vi "CRYGet Tab Reference.vi"(10 "Label Name":string, 11 "VI Refnum":refnum<vi>) -> (1 "Find?":bool, 2 "Tab Ref Out":refnum<vi>, 3 "VI Refnum Out":refnum<vi>)   [LabVIEW 2013]
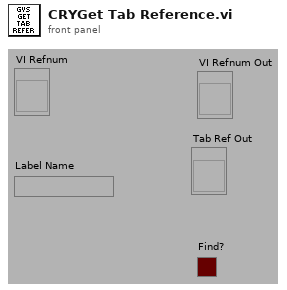
[diagram p1: front panel]
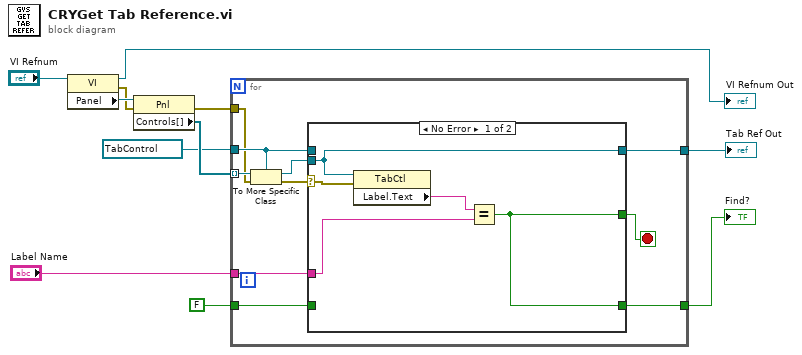
[diagram p0: block diagram]
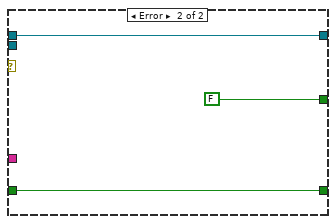
[diagram p2: hidden frame]
diagram:
  n1 = property class="VI"(reference="VI Refnum") -> (reference out=→"VI Refnum Out":refnum<vi>, error out=w2:errorcluster, "Panel"=w6:refnum<vi>)  [unwired: 1 in]
  n2 = property class="Pnl"(reference=w6, error in=w2) -> (error out=w1:errorcluster, "Controls[]"=w10:refnum<vi>[])  [unwired: 1 out]
  n3 = for {
    tunnel: w10 -> [w21] mode=indexing
    tunnel: [w17] -> w3
    tunnel: "Label Name" -> [w16]
    tunnel: refnum<vi> refnum ("Tab Control") -> [w15]
    tunnel: FALSE ("Boolean") -> [w14]
    tunnel: [w13] -> w7
    tunnel: w1 -> [w12]
    stop <- w18 stop-if-true
    n4 = To More Specific Class(target class=w15, reference=w21, error in=w12) -> (specific class reference=w19:refnum<vi>, error out=w20:errorcluster)
    n5 = case shown="No Error" w20 {
      selector: w20 -> [w22 _]
      tunnel: w19 -> [w24 _]
      tunnel: [w23 FALSE] -> w18
      tunnel: [w24 w28] -> w17
      tunnel: w16 -> [w25 _]
      tunnel: w15 -> [_ w28]
      tunnel: [w23 w27] -> w13
      tunnel: w14 -> [_ w27]
      frame No Error {
        n6 = property class="TabCtl"(reference=w24, error in=w22) -> ("Label.Text"=w26:string)  [unwired: 2 out]
        n7 = Equal?(x=w26, y=w25) -> (x = y?=w23:bool)
      }
      frame Error {
      }
    }
  }
  "Find?" <- w7
  "Tab Ref Out" <- w3
